vi "DB_LeeEventos.vi"() -> (0 "error out":errorcluster, 3 "eventos out":string)   [LabVIEW 2018]
uses:
  <vilib>/addons/database/Connection.llb/DB Tools Open Connec (Path).vi
  <vilib>/addons/database/Connection.llb/Conn Execute.vi
  <vilib>/addons/database/Recordset.llb/Rec Fetch Recordset Data (R).vi
  <vilib>/addons/database/Recordset.llb/Rec Destroy - Connection.vi
  <vilib>/addons/database/_DB Variant To Data/Database Variant To Data.xnode
  <vilib>/addons/database/NI_Database_API.lvlib
panel:
  out "5 min atras":string
  out "fecha actual":string
  in  "error in (no error)":errorcluster
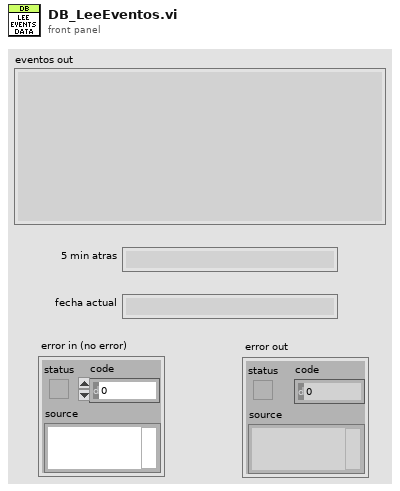
[diagram p1: front panel]
types:
  T1 = typedef "NI_Database_API.lvlib/Conn ObjectReference.ctl" = refnum<k1>
  T2 = typedef "NI_Database_API.lvlib/Rec ObjectReference.ctl" = refnum<k1>
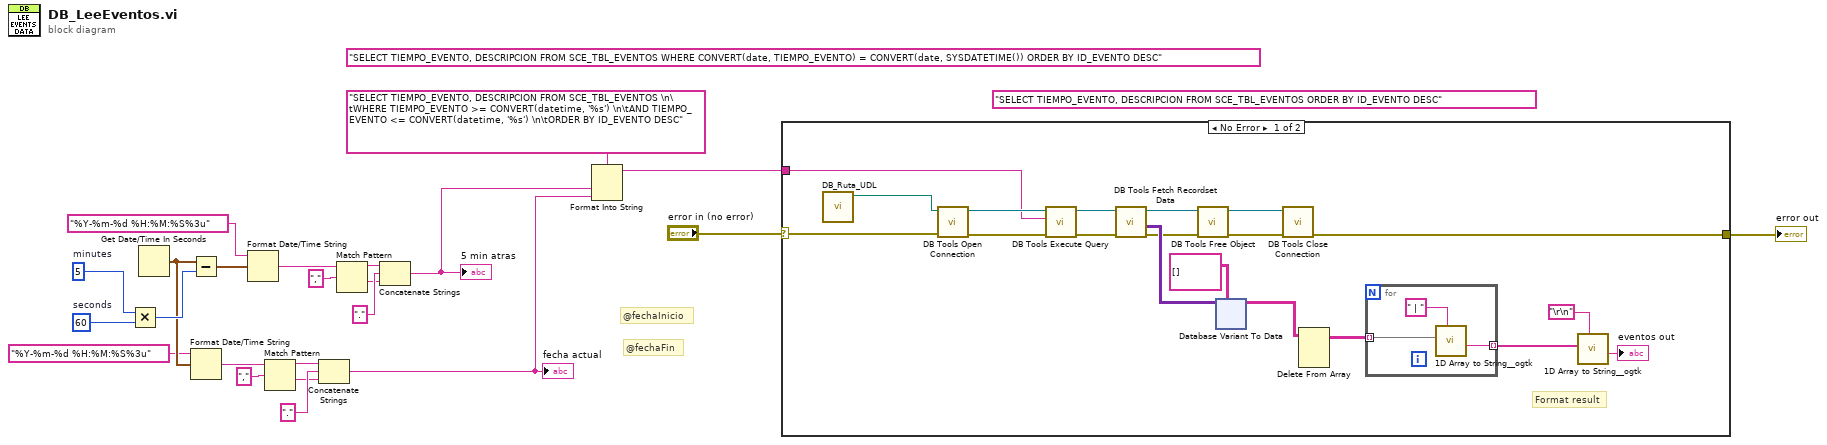
[diagram p0: block diagram]
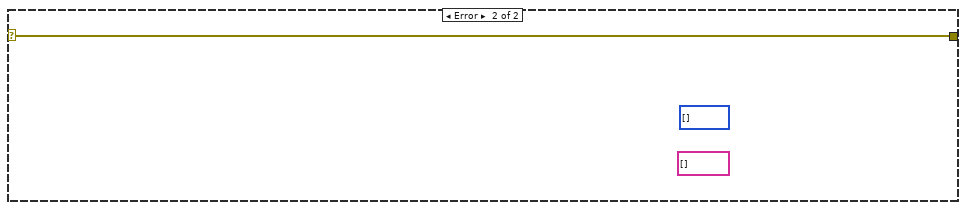
[diagram p2: hidden frame]
diagram:
  w16 = 60  # seconds
  w15 = 5  # minutes
  (unwired) "SELECT TIEMPO_EVENTO, DESCRIPCION FROM SCE_TBL_EVENTOS WHERE CONVERT(date, TIEMPO_EVENTO) = CONVERT(date, SYSDATETIME()) ORDER BY ID_EVENTO DESC" ("SQL")
  (unwired) "SELECT TIEMPO_EVENTO, DESCRIPCION FROM SCE_TBL_EVENTOS ORDER BY ID_EVENTO DESC" ("SQL")
  # "@fechaFin"
  # "@fechaInicio"
  n1 = Multiply(x=w15, y=w16) -> (x*y=w17:i32)
  n2 = Get Date/Time In Seconds() -> (seconds since 1Jan1904=w14:timestamp)
  n3 = Subtract(x=w14, y=w17) -> (x-y=w19:timestamp)
  n4 = Format Date/Time String(time format string (%c)="%Y-%m-%d %H:%M:%S%3u", seconds (now)=w14) -> (date/time string=w6:string)  [unwired: 1 in]
  n5 = Format Date/Time String(time format string (%c)="%Y-%m-%d %H:%M:%S%3u", seconds (now)=w19) -> (date/time string=w12:string)  [unwired: 1 in]
  n6 = Match Pattern(string=w6, regular expression=",") -> (before substring=w4:string, after substring=w3:string)  [unwired: 1 in, 2 out]
  n7 = Concatenate Strings(w4, "." ("string"), w3) -> (w1:string)
  "fecha actual" <- w1
  n8 = Match Pattern(string=w12, regular expression=",") -> (before substring=w10:string, after substring=w8:string)  [unwired: 1 in, 2 out]
  n9 = Concatenate Strings(w10, "." ("string"), w8) -> (w2:string)
  "5 min atras" <- w2
  n10 = Format Into String(format string="SELECT TIEMPO_EVENTO, DESCRIPCION FROM SCE_TBL_EVENTOS \n\tWHERE TIEMPO_EVENTO >= CONVERT(datetime, '%s') \n\tAND TIEMPO_EVENTO <= CONVERT(datetime, '%s') \n\tORDER BY ID_EVENTO DESC" ("SQL"), w2, w1) -> (resulting string=w20:string)  [unwired: 2 in, 1 out]
  n11 = case shown="No Error" "error in (no error)" {
    selector: "error in (no error)" -> [w37 w90]
    tunnel: [w39 w90] -> w23
    tunnel: w20 -> [w36 _]
    frame No Error {
      # "Format result"
      n12 = call "DB_Ruta_UDL.vi"() -> ("UDL ruta"=w25:path)  [unwired: 11 in]
      n13 = call-poly <vilib>:"DB Tools Open Connection.vi"("error in (no error)"=w37, "connection information"=w25) -> ("error out"=w42:errorcluster, "connection reference"=w40:T1)  [unwired: 6 in]
      n14 = call-poly <vilib>:"DB Tools Execute Query.vi"("error in (no error)"=w42, "SQL query"=w36, "connection reference"=w40) -> ("error out"=w38:errorcluster, "recordset reference"=w35:T2)  [unwired: 5 in]
      n15 = call-poly <vilib>:"DB Tools Fetch Recordset Data.vi"("error in (no error)"=w38, "recordset reference"=w35) -> ("error out"=w31:errorcluster, "recordset data"=w32:variant[][], "recordset reference out"=w34:T2)  [unwired: 3 in]
      n16 = call-poly <vilib>:"DB Tools Free Object.vi"("error in (no error)"=w31, "recordset reference"=w34) -> ("error out"=w41:errorcluster, "connection reference"=w24:T1)  [unwired: 8 in]
      n17 = xnode "Database Variant To Data"("database variant"=w32, "type"=string[][] []) -> ("data"=w30:string[][])  [unwired: 1 in, 1 out]
      n18 = call <vilib>:"DB Tools Close Connection.vi"("error in (no error)"=w41, "connection reference"=w24) -> ("error out"=w39:errorcluster)  [unwired: 5 in]
      n19 = Delete From Array(array=w30) -> (array with subset deleted=w27:string[][])  [unwired: 3 in, 1 out]
      n20 = for {
        tunnel: w27 -> [w45] mode=indexing
        tunnel: [w44] -> w29 mode=indexing
        n21 = call <userlib>:"1D Array to String__ogtk.vi"("delimiter (Tab)"=" | ", "Array of Strings"=w45) -> ("delimited string"=w44:string)  [unwired: 9 in]
      }
      n22 = call <userlib>:"1D Array to String__ogtk.vi"("delimiter (Tab)"="\r\n", "Array of Strings"=w29) -> ("delimited string"=→"eventos out":string)  [unwired: 9 in]
    }
    frame Error {
      (unwired) string[] [] ("data")
      (unwired) i32[] []
    }
  }
  "error out" <- w23
